vi "TestLidar.vi"() -> ()   [LabVIEW 2016]
panel:
  out "Measurement Data":i32[](array[numeric])
  out "XY Graph":cluster{dbl[], dbl[]}[](graph)
  in  "Stop":bool
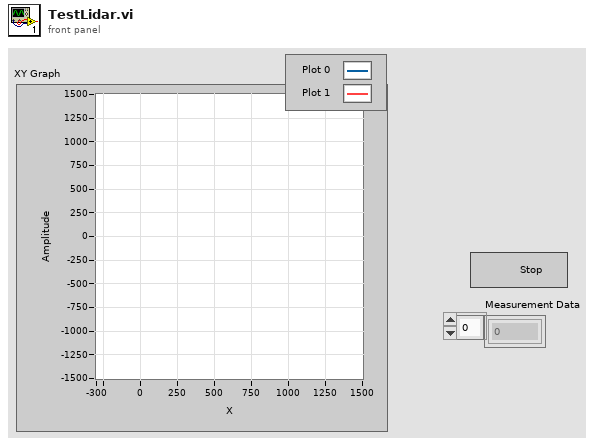
[diagram p1: front panel]
types:
  T1 = typedef "Measurement Parameters.ctl" = cluster{"Start Step":u32, "End Step":u32, "Cluster Count":u32, "Scan Interval":u32, "Number of Scans":u32, "Measurement Type":T2}
  T2 = typedef "Measurement Type.ctl" = enum16{"MS"}
  T3 = cluster{"x_norm":dbl, "y_norm":dbl, "x LiDAR":dbl[], "y LiDAR":dbl[]}
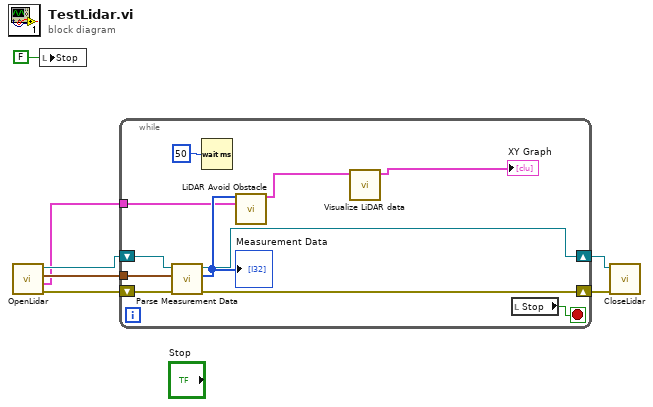
[diagram p0: block diagram]
diagram:
  n1 = call "OpenLidar.vi"() -> ("error out"=w6:errorcluster, "Params Out"=w1:cluster{"angle":dbl[], "id":i32[], "kk":dbl[]}, "Measurement Parameters"=w2:T1, "VISA Refnum out"=w7:refnum<visa-resource-name>)  [unwired: 8 in]
  n2 = local write "Stop"(FALSE ("Stop")) -> ()
  n3 = while {
    tunnel: w2 -> [w16]
    shift-right: [w12] -> w5
    shift-left: w7 -> [w15]
    shift-right: [w13] -> w4
    shift-left: w6 -> [w14]
    tunnel: w1 -> [w10]
    stop <- w17 stop-if-true
    n4 = call "Parse Measurement Data.vi"("error in (no error)"=w14, "Measurement Parameters"=w16, "VISA Refnum in"=w15) -> ("error out"=w13:errorcluster, "Measurement Data"=w11:i32[], "VISA Refnum out"=w12:refnum<visa-resource-name>)  [unwired: 6 in]
    "Measurement Data" <- w11
    n5 = Wait (ms)(milliseconds to wait=u32 50) -> ()  [unwired: 1 out]
    n6 = call "LiDAR Avoid Obstacle.vi"("Measurement Data"=w11, "Input Params"=w10) -> ("Output data"=w9:T3)  [unwired: 12 in, 1 out]
    n7 = call "Visualize LiDAR data.vi"("Input LiDAR"=w9) -> ("Array"=→"XY Graph":cluster{"x LiDAR":dbl[], "y LiDAR":dbl[]}[])  [unwired: 10 in]
    n8 = local read "Stop"() -> (w17:bool)
  }
  n9 = call "CloseLidar.vi"("error in (no error)"=w4, "VISA Refnum in"=w5) -> ()  [unwired: 10 in]
